vi "ModelCode_Rf3.vi"(9 "BarCode":string, 11 "Data In":T1) -> (1 "ModeCode":string, 3 "Data Out":T1)   [LabVIEW 2014]
uses:
  controls/Data.ctl
panel:
  # "日期"
  # "機種名稱"
  # "機種代號"
  # "商品條碼"
  # "台"
  # "OK"
  # "NG"
  # "台"
  # "總計"
  # "台"
  # "日期"
  # "機種名稱"
  # "機種代號"
  # "商品條碼"
  # "台"
  # "OK"
  # "NG"
  # "台"
  # "總計"
  # "台"
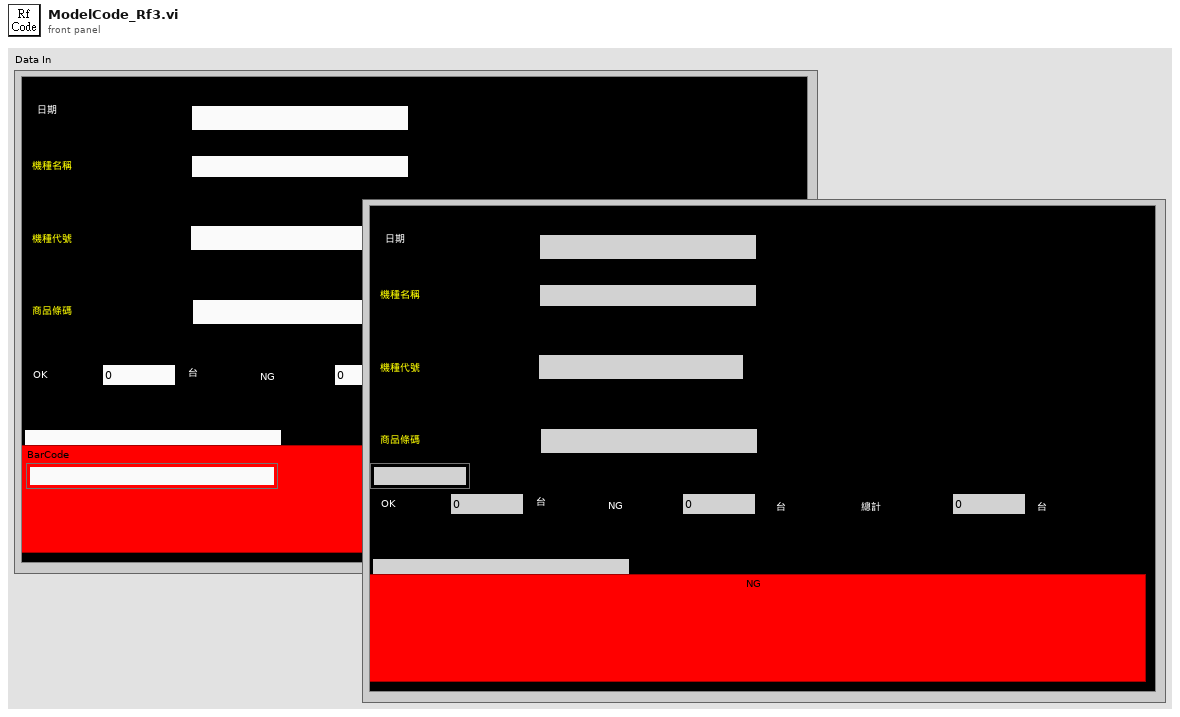
[diagram p1: front panel]
types:
  T1 = typedef "Data.ctl" = cluster{"Date":string, "BarCode1":string, "BarCode2":string, "BarCode3":string, "Message":string, "OK Count":u16, "NG Count":u16, "Total Count":u16, "ModelData":string[][], "OK&NG":bool, "COM1":refnum<visa-resource-name>, "COM2":refnum<visa-resource-name>, "IO":i32, "Time":u32, "TCP":refnum<k5>, "TCP 2":refnum<k5>}
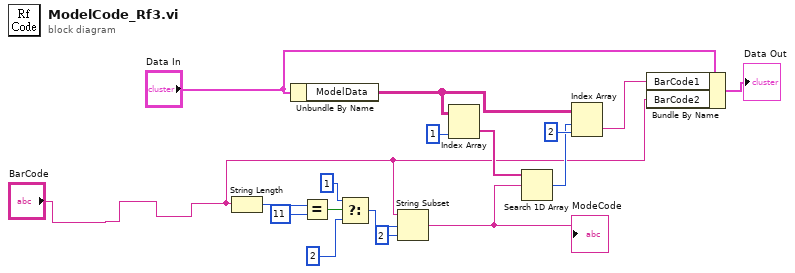
[diagram p0: block diagram]
diagram:
  n1 = String Length(string="BarCode") -> (length=w17:i32)
  n2 = Unbundle By Name("Data In") -> ("ModelData"=w7:string[][])
  n3 = Equal?(x=w17, y=11) -> (x = y?=w15:bool)
  n4 = Select(t=1 ("offset (0)"), s=w15, f=2) -> (s? t:f=w13:i32)
  n5 = String Subset(string="BarCode", offset (0)=w13, length (rest)=2 ("length (rest)")) -> (substring=w8:string)
  "ModeCode" <- w8
  n6 = Index Array(array=w7, index (col)=1 ("disabled index (col)")) -> (element=w9:string[])  [unwired: 1 in]
  n7 = Search 1D Array(1D array=w9, element=w8) -> (index of element=w5:i32)  [unwired: 1 in]
  n8 = Index Array(array=w7, index (row)=w5, index (col)=2 ("disabled index (col)")) -> (element=w2:string)
  n9 = Bundle By Name(cluster="Data In", "BarCode1"=w2, "BarCode2"="BarCode") -> (→"Data Out":T1)
